vi "Update an Attribute.vi"(0 "attributes in":variant, 5 "error in (no error)":errorcluster, 6 "Attribute List":T1, 7 "Attribute Value":string, 8 "Attribute Option":T2) -> (14 "attributes out":variant, 19 "error out":errorcluster)   [LabVIEW 2020, in "GSwFormDSP.lvclass"]
uses:
  GSwFormDSP.lvclass
  functions/Attribute Options.ctl
  functions/Attribute List.ctl
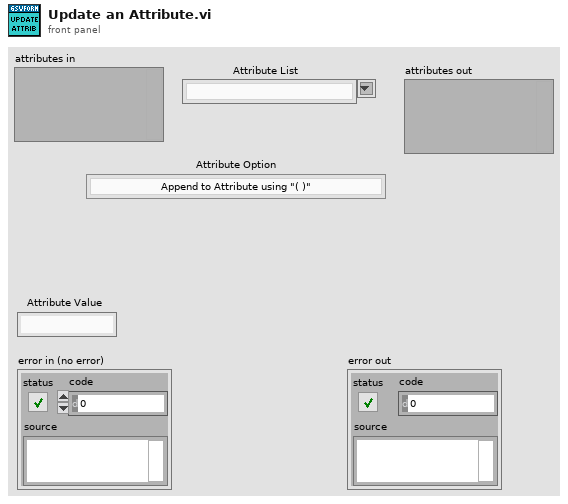
[diagram p1: front panel]
types:
  T1 = typedef "GSwFormDSP.lvclass/Attribute List.ctl" = string
  T2 = typedef "GSwFormDSP.lvclass/Attribute Options.ctl" = enum16{"Append to Attribute using \"( )\"", "Replace Attribute Value"}
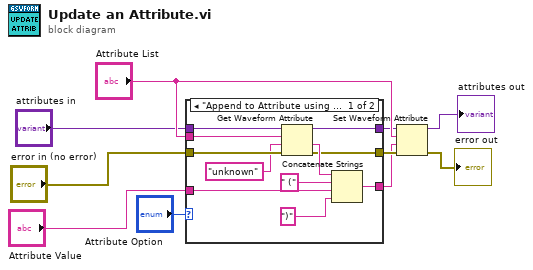
[diagram p0: block diagram]
diagram:
  n1 = case shown="\"Append to Attribute using \\\"( )\\\"\", Default" "Attribute Option" {
    tunnel: "attributes in" -> [w21 w22]
    tunnel: "error in (no error)" -> [w20 w23]
    tunnel: [w15 w22] -> w4
    tunnel: "Attribute List" -> [w14 _]
    tunnel: [w13 w24] -> w6
    tunnel: [w12 w23] -> w7
    tunnel: "Attribute Value" -> [w11 w24]
    frame "Append to Attribute using \"( )\"", Default {
      n2 = Get Waveform Attribute(4:w20, 5:"unknown", 6:w14, 7:w21) -> (0:w12:errorcluster, 1:w18:string, 3:w15:variant)  [unwired: 1 out]
      n3 = Concatenate Strings(w18, " (" ("string"), w11, ")") -> (w13:string)
    }
    frame "Replace Attribute Value" {
    }
  }
  n4 = Set Waveform Attribute(4:w7, 5:w6, 6:"Attribute List", 7:w4) -> (0:→"error out":errorcluster, 3:→"attributes out":variant)  [unwired: 1 out]
